vi "ClusterToDescriptiveString.vi"(8 "error in":errorcluster, 11 "Cluster In":refnum<vi>) -> (0 "error out":errorcluster, 3 "String":string)   [LabVIEW 2023]
doc: "This VI turns a <b>cluster</b> (from reference) into a human/machine readable <b>string</b>.\n\n<b>Cluster in</b> - A reference to the cluster to describe. \n<b>String</b> - Description string out"
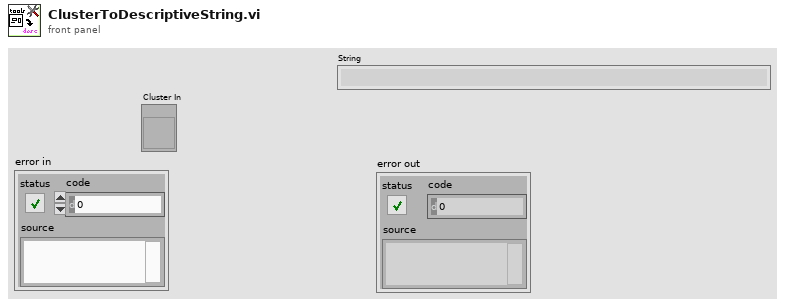
[diagram p1: front panel]
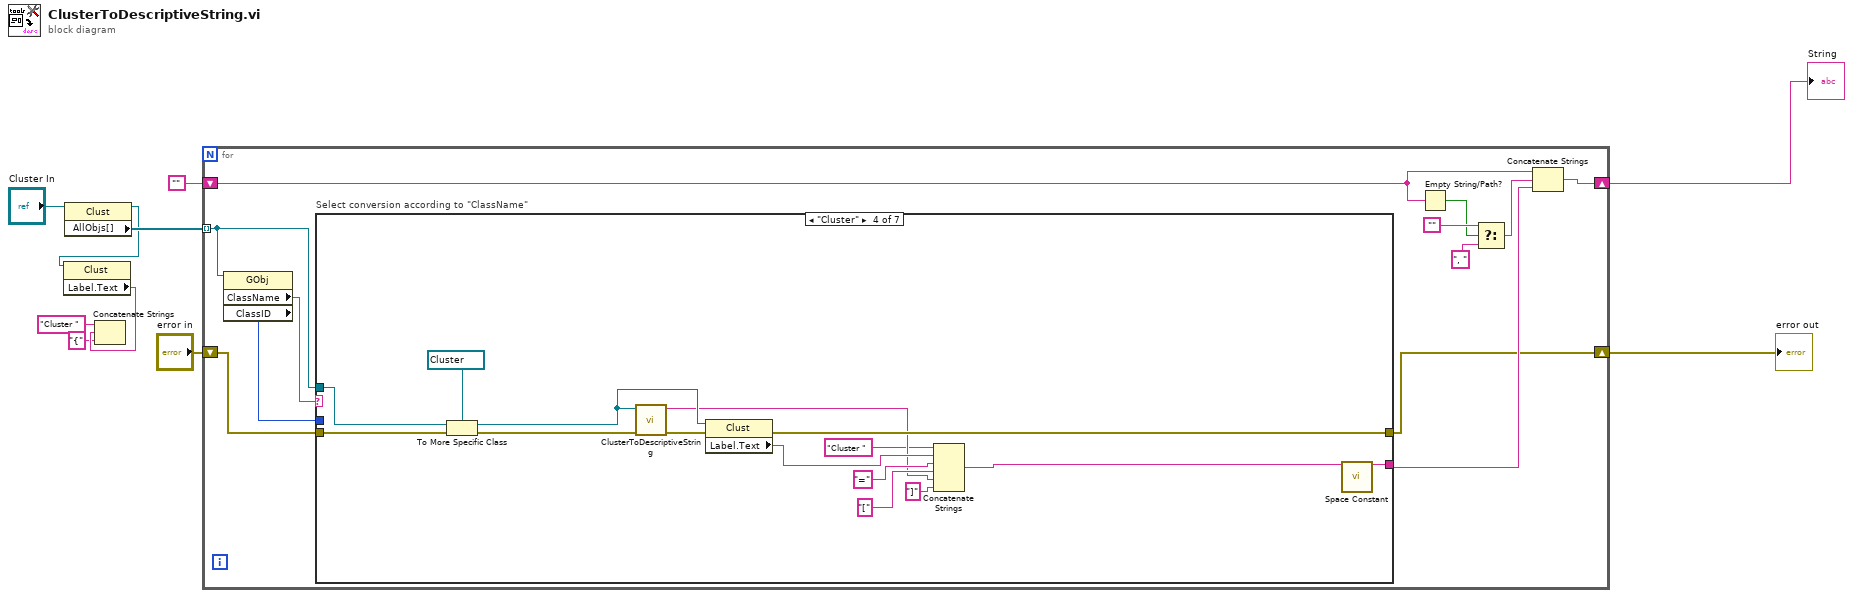
[diagram p0: block diagram]
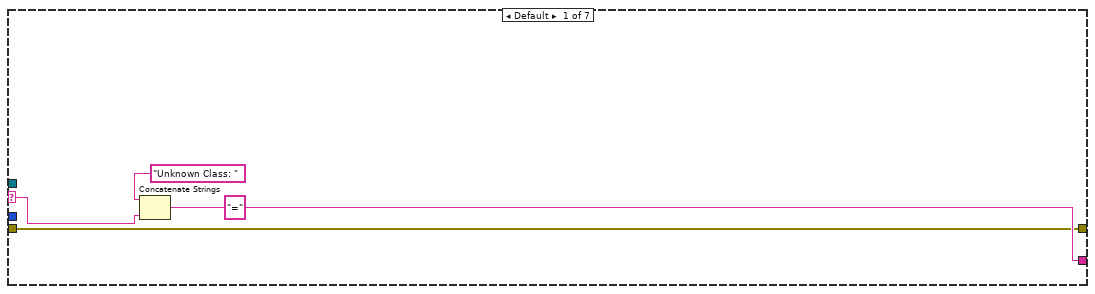
[diagram p2: hidden frame]
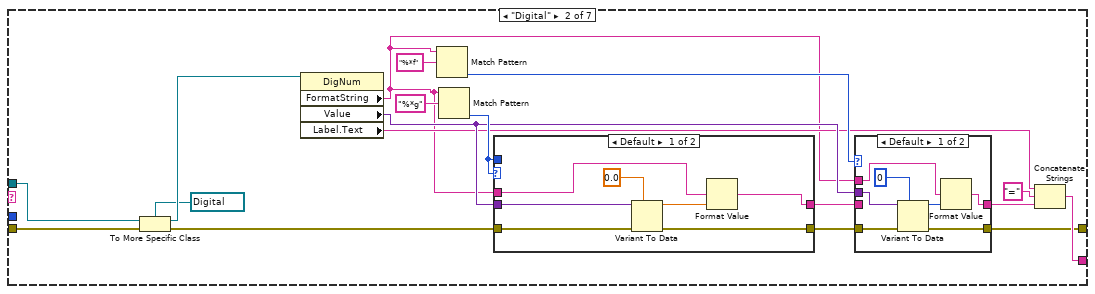
[diagram p3: hidden frame]
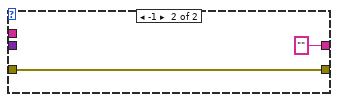
[diagram p5: hidden frame]
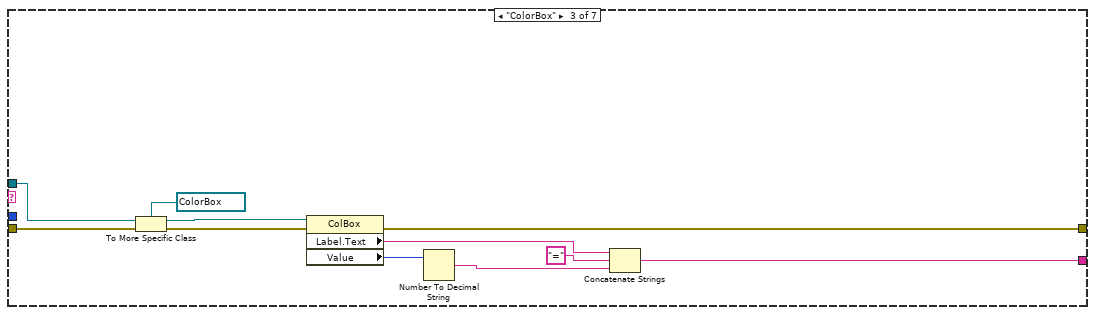
[diagram p6: hidden frame]
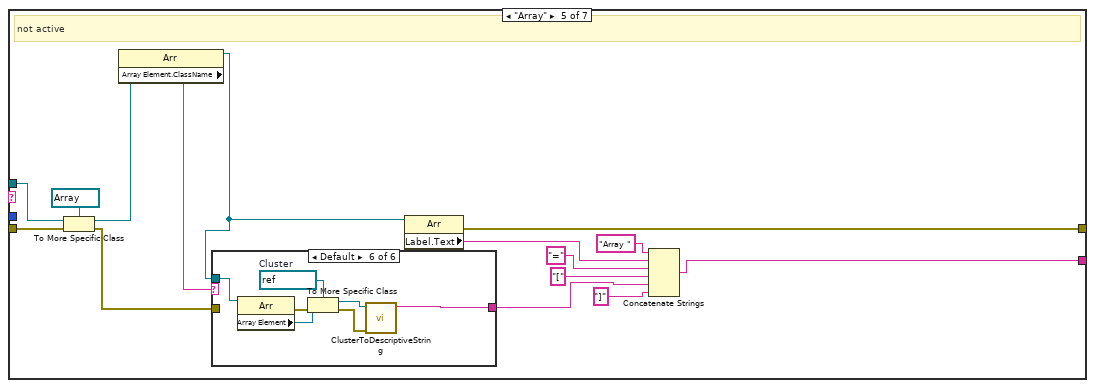
[diagram p7: hidden frame]
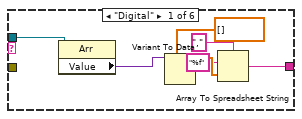
[diagram p8: hidden frame]
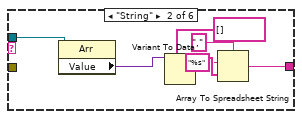
[diagram p9: hidden frame]
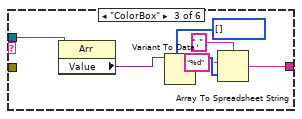
[diagram p10: hidden frame]
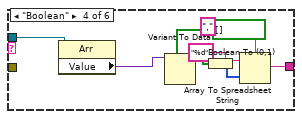
[diagram p11: hidden frame]
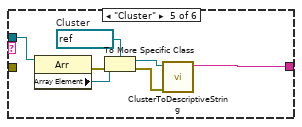
[diagram p12: hidden frame]
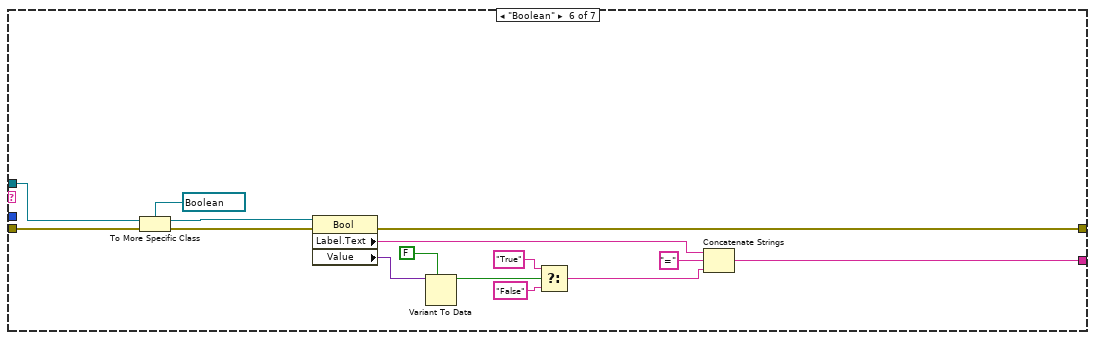
[diagram p13: hidden frame]
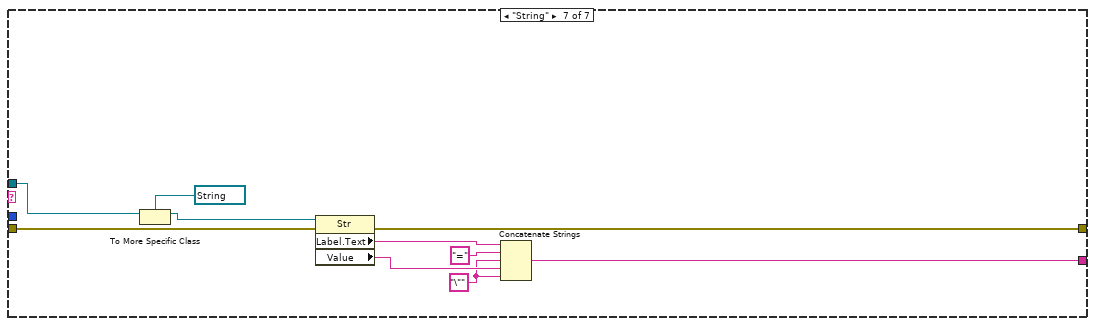
[diagram p14: hidden frame]
diagram:
  n1 = property on="Property Node" class="Clust"(reference="Cluster In") -> (reference out=w4:refnum<vi>, "AllObjs[]"=w6:refnum<vi>[])  [unwired: 1 in, 1 out]
  n2 = property on="Property Node" class="Clust"(reference=w4) -> ("Label.Text"=w2:string)  [unwired: 1 in, 2 out]
  n3 = Concatenate Strings("Cluster " ("string"), w2, "{" ("string")) -> ()  [unwired: 1 out]
  n4 = for {
    tunnel: w6 -> [w21] mode=indexing
    shift-right: [w22] -> w10
    shift-left: "" ("Empty String Constant") -> [w12]
    shift-right: [w15] -> w7
    shift-left: "error in" -> [w14]
    n5 = property on="Property Node" class="GObj"(reference=w21) -> ("ClassName"=w19:string, "ClassID"=w20:u32)  [unwired: 1 in, 2 out]
    n6 = case "Select conversion according to \"ClassName\"" shown="\"Cluster\"" w19 {
      selector: w19 -> [w25 _ _ _ _ _ _]
      tunnel: [w24 w35 w70 w86 w101 w158 w169] -> w18
      tunnel: w21 -> [_ w45 w74 w88 w103 w161 w171]
      tunnel: w20 -> [_ _ _ _ _ _ _]
      tunnel: [w23 w29 w66 w83 w99 w149 w163] -> w15
      tunnel: w14 -> [w23 w32 w64 w82 w98 w147 w162]
      frame Default {
        n7 = Concatenate Strings("Unknown Class: ", "=", w25) -> (w24:string)
      }
      frame "Digital" {
        n8 = To More Specific Class(target class=refnum<vi> refnum ("567"), reference=w45, error in=w32) -> (specific class reference=w44:refnum<vi>, error out=w31:errorcluster)
        n9 = property on="Property Node" class="DigNum"(reference=w44) -> ("FormatString"=w34:string, "Value"=w41:variant, "Label.Text"=w37:string)  [unwired: 1 in, 2 out]
        n10 = Match Pattern(string=w34, regular expression="%*f") -> (offset past match=w38:i32)  [unwired: 1 in, 3 out]
        n11 = Match Pattern(string=w34, regular expression="%*g") -> (offset past match=w43:i32)  [unwired: 1 in, 3 out]
        n12 = case shown="Default" w43 {
          tunnel: w43 -> [_ _]
          tunnel: w41 -> [w61 _]
          tunnel: [w59 "" ("output string")] -> w42
          tunnel: w34 -> [w58 _]
          tunnel: w31 -> [w57 w62]
          tunnel: [w56 w62] -> w30
          frame Default {
            n13 = Variant To Data(error in=w57, type=0.0, Variant=w61) -> (data=w60:dbl, error out=w56:errorcluster)
            n14 = Format Value(format string=w58, value (0)=w60) -> (output string=w59:string)  [unwired: 1 in]
          }
          frame -1 {
          }
        }
        n15 = case shown="Default" w38 {
          tunnel: w41 -> [w52 _]
          tunnel: w42 -> [_ w54]
          tunnel: [w50 w54] -> w36
          tunnel: w34 -> [w49 _]
          tunnel: w30 -> [w48 w53]
          tunnel: [w47 w53] -> w29
          frame Default {
            n16 = Variant To Data(error in=w48, type=0, Variant=w52) -> (data=w51:i32, error out=w47:errorcluster)
            n17 = Format Value(format string=w49, value (0)=w51) -> (output string=w50:string)  [unwired: 1 in]
          }
          frame -1 {
          }
        }
        n18 = Concatenate Strings(w37, "=" ("string"), w36) -> (w35:string)
      }
      frame "ColorBox" {
        n19 = To More Specific Class(target class=refnum<vi> refnum ("Left"), reference=w74, error in=w64) -> (specific class reference=w73:refnum<vi>, error out=w65:errorcluster)
        n20 = property on="Property Node" class="ColBox"(reference=w73, error in=w65) -> (error out=w66:errorcluster, "Label.Text"=w71:string, "Value"=w68:u32)  [unwired: 1 out]
        n21 = Number To Decimal String(number=w68) -> (decimal integer string=w72:string)  [unwired: 1 in]
        n22 = Concatenate Strings(w71, "=" ("string"), w72) -> (w70:string)
      }
      frame "Cluster" {
        n23 = To More Specific Class(target class=refnum<vi> refnum ("Left"), reference=w88, error in=w82) -> (specific class reference=w80:refnum<vi>, error out=w81:errorcluster)
        n24 = call "ClusterToDescriptiveString.vi"("error in"=w81, "Cluster In"=w80) -> ("error out"=w79:errorcluster, "String"=w77:string)  [unwired: 8 in]
        n25 = property on="Property Node" class="Clust"(reference=w80, error in=w79) -> (error out=w83:errorcluster, "Label.Text"=w87:string)  [unwired: 1 out]
        n26 = Concatenate Strings("Cluster " ("string"), w87, "=" ("string"), "[" ("string"), w77, "]" ("string")) -> (w86:string)
        n27 = call <vilib>:"Space Constant.vi"() -> ()  [unwired: 1 out]
      }
      frame "Array" {
        # "not active"
        n28 = To More Specific Class(target class=refnum<vi> refnum ("Left"), reference=w103, error in=w98) -> (specific class reference=w93:refnum<vi>, error out=w89:errorcluster)
        n29 = property on="Property Node" class="Arr"(reference=w93) -> (reference out=w91:refnum<vi>, "Array Element.ClassName"=w92:string)  [unwired: 1 in, 1 out]
        n30 = case shown="Default" w92 {
          tunnel: w91 -> [w110 w117 w124 w132 w139 w146]
          tunnel: [w106 w113 w120 w125 w135 w142] -> w90
          tunnel: w89 -> [_ _ _ _ _ _]
          frame "Digital" {
            n31 = property on="Property Node" class="Arr"(reference=w110) -> ("Value"=w109:variant)  [unwired: 1 in, 2 out]
            n32 = Variant To Data(type=dbl[] [], Variant=w109) -> (data=w107:dbl[])  [unwired: 1 in, 1 out]
            n33 = Array To Spreadsheet String(delimiter (Tab)=",", array=w107, 3:"%f" ("format string")) -> (spreadsheet string=w106:string)
          }
          frame "String" {
            n34 = property on="Property Node" class="Arr"(reference=w117) -> ("Value"=w116:variant)  [unwired: 1 in, 2 out]
            n35 = Variant To Data(type=string[] [], Variant=w116) -> (data=w114:string[])  [unwired: 1 in, 1 out]
            n36 = Array To Spreadsheet String(delimiter (Tab)=",", array=w114, 3:"%s" ("format string")) -> (spreadsheet string=w113:string)
          }
          frame "ColorBox" {
            n37 = property on="Property Node" class="Arr"(reference=w124) -> ("Value"=w123:variant)  [unwired: 1 in, 2 out]
            n38 = Variant To Data(type=u32[] [], Variant=w123) -> (data=w121:u32[])  [unwired: 1 in, 1 out]
            n39 = Array To Spreadsheet String(delimiter (Tab)=",", array=w121, 3:"%d" ("format string")) -> (spreadsheet string=w120:string)
          }
          frame "Boolean" {
            n40 = property on="Property Node" class="Arr"(reference=w132) -> ("Value"=w131:variant)  [unwired: 1 in, 2 out]
            n41 = Variant To Data(type=bool[] [], Variant=w131) -> (data=w129:bool[])  [unwired: 1 in, 1 out]
            n42 = Boolean To (0,1)(Boolean=w129) -> (0, 1=w128:i16[])
            n43 = Array To Spreadsheet String(delimiter (Tab)=",", array=w128, 3:"%d" ("format string")) -> (spreadsheet string=w125:string)
          }
          frame "Cluster" {
            w137 = refnum<vi> refnum  # Cluster
            n44 = property class="Arr"(reference=w139) -> (error out=w133:errorcluster, "Array Element"=w138:refnum<vi>)  [unwired: 1 in, 1 out]
            n45 = To More Specific Class(target class=w137, reference=w138, error in=w133) -> (specific class reference=w136:refnum<vi>, error out=w134:errorcluster)
            n46 = call "ClusterToDescriptiveString.vi"("error in"=w134, "Cluster In"=w136) -> ("String"=w135:string)  [unwired: 8 in, 1 out]
          }
          frame Default {
            w144 = refnum<vi> refnum  # Cluster
            n47 = property class="Arr"(reference=w146) -> (error out=w140:errorcluster, "Array Element"=w145:refnum<vi>)  [unwired: 1 in, 1 out]
            n48 = To More Specific Class(target class=w144, reference=w145, error in=w140) -> (specific class reference=w143:refnum<vi>, error out=w141:errorcluster)
            n49 = call "ClusterToDescriptiveString.vi"("error in"=w141, "Cluster In"=w143) -> ("String"=w142:string)  [unwired: 8 in, 1 out]
          }
        }
        n50 = property on="Property Node" class="Arr"(reference=w91) -> (error out=w99:errorcluster, "Label.Text"=w102:string)  [unwired: 1 in, 1 out]
        n51 = Concatenate Strings("Array " ("string"), w102, "=" ("string"), "[" ("string"), w90, "]" ("string")) -> (w101:string)
      }
      frame "Boolean" {
        n52 = To More Specific Class(target class=refnum<vi> refnum ("Left"), reference=w161, error in=w147) -> (specific class reference=w160:refnum<vi>, error out=w148:errorcluster)
        n53 = property on="Property Node" class="Bool"(reference=w160, error in=w148) -> (error out=w149:errorcluster, "Label.Text"=w159:string, "Value"=w155:variant)  [unwired: 1 out]
        n54 = Variant To Data(type=FALSE ("x = y?"), Variant=w155) -> (data=w153:bool)  [unwired: 1 in, 1 out]
        n55 = Select(t="True" ("Label.Text"), s=w153, f="False" ("Label.Text")) -> (s? t:f=w150:string)
        n56 = Concatenate Strings(w159, "=" ("string"), w150) -> (w158:string)
      }
      frame "String" {
        w166 = "\"" ("string")
        n57 = To More Specific Class(target class=refnum<vi> refnum ("Numeric"), reference=w171) -> (specific class reference=w170:refnum<vi>)  [unwired: 1 in, 1 out]
        n58 = property on="Property Node" class="Str"(reference=w170, error in=w162) -> (error out=w163:errorcluster, "Label.Text"=w165:string, "Value"=w167:string)  [unwired: 1 out]
        n59 = Concatenate Strings(w165, "=" ("string"), w166, w167, w166) -> (w169:string)
      }
    }
    n60 = Empty String/Path?(string/path=w12) -> (empty?=w11:bool)
    n61 = Select(t="" ("Empty String Constant"), s=w11, f=", " ("string")) -> (s? t:f=w16:string)
    n62 = Concatenate Strings(w12, w16, w18) -> (w22:string)
  }
  "String" <- w10
  "error out" <- w7
